vi "Read Scale Range.vi"(8 "error in (no error)":errorcluster, 11 "Ctl Refnum in":refnum<vi>) -> (0 "error out":errorcluster, 1 "Max":dbl, 2 "Min":dbl, 3 "Ctl Refnum":refnum<vi>)   [LabVIEW 2020, in "VolatusGUIEditorCore.lvlib"]
uses:
  VolatusGUIEditorCore.lvlib
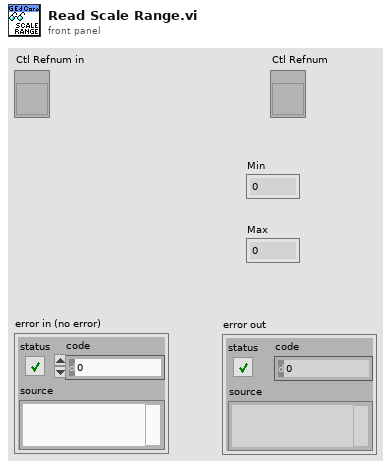
[diagram p1: front panel]
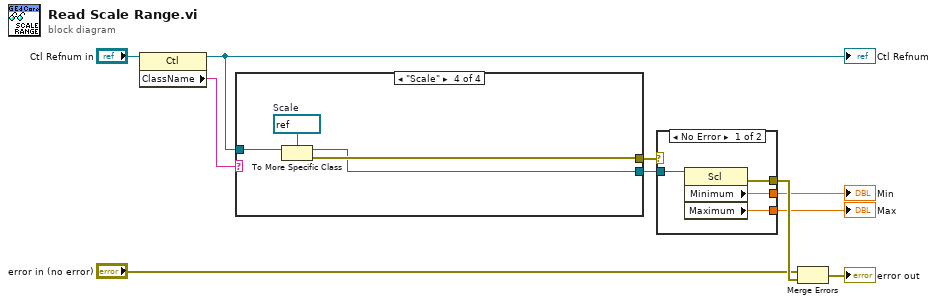
[diagram p0: block diagram]
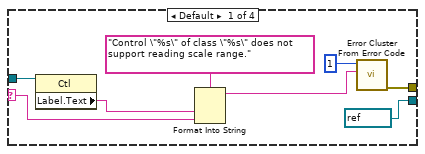
[diagram p2: hidden frame]
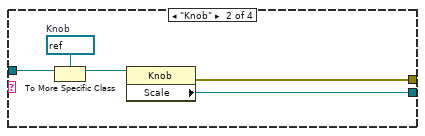
[diagram p3: hidden frame]
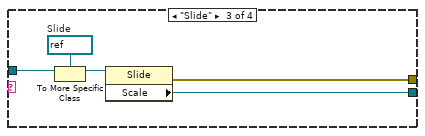
[diagram p4: hidden frame]
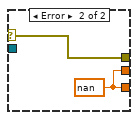
[diagram p5: hidden frame]
diagram:
  n1 = property class="Ctl"(reference="Ctl Refnum in") -> (reference out=w7:refnum<vi>, "ClassName"=w8:string)  [unwired: 1 in, 1 out]
  "Ctl Refnum" <- w7
  n2 = case shown="\"Scale\"" w8 {
    selector: w8 -> [w15 _ _ _]
    tunnel: w7 -> [w18 w23 w28 w32]
    tunnel: [refnum<vi> refnum ("Scale") w19 w25 w29] -> w4
    tunnel: [w13 w20 w24 w30] -> w1
    frame Default {
      n3 = property class="Ctl"(reference=w18) -> ("Label.Text"=w16:string)  [unwired: 1 in, 2 out]
      n4 = Format Into String(format string="Control \"%s\" of class \"%s\" does not support reading scale range.", w16, w15) -> (resulting string=w14:string)  [unwired: 2 in, 1 out]
      n5 = call <vilib>:"Error Cluster From Error Code.vi"("error message (\"\")"=w14, "error code (0)"=1) -> ("error out"=w13:errorcluster)  [unwired: 7 in]
    }
    frame "Knob" {
      w22 = refnum<vi> refnum  # Knob
      n6 = To More Specific Class(target class=w22, reference=w23) -> (specific class reference=w21:refnum<vi>)  [unwired: 1 in, 1 out]
      n7 = property class="Knob"(reference=w21) -> (error out=w20:errorcluster, "Scale"=w19:refnum<vi>)  [unwired: 1 in, 1 out]
    }
    frame "Slide" {
      w27 = refnum<vi> refnum  # Slide
      n8 = To More Specific Class(target class=w27, reference=w28) -> (specific class reference=w26:refnum<vi>)  [unwired: 1 in, 1 out]
      n9 = property class="Slide"(reference=w26) -> (error out=w24:errorcluster, "Scale"=w25:refnum<vi>)  [unwired: 1 in, 1 out]
    }
    frame "Scale" {
      w31 = refnum<vi> refnum  # Scale
      n10 = To More Specific Class(target class=w31, reference=w32) -> (specific class reference=w29:refnum<vi>, error out=w30:errorcluster)  [unwired: 1 in]
    }
  }
  n11 = case shown="No Error" w1 {
    selector: w1 -> [_ w38]
    tunnel: w4 -> [w36 _]
    tunnel: [w35 w37] -> w3
    tunnel: [w34 w37] -> w2
    tunnel: [w33 w38] -> w10
    frame No Error {
      n12 = property class="Scl"(reference=w36) -> (error out=w33:errorcluster, "Minimum"=w35:dbl, "Maximum"=w34:dbl)  [unwired: 1 in, 1 out]
    }
    frame Error {
      w37 = nan ("Maximum")
    }
  }
  "Min" <- w3
  "Max" <- w2
  n13 = Merge Errors("error in (no error)", w10) -> (→"error out":errorcluster)
